vi "Entry.vi"(8 "error in (no error)":errorcluster, 11 "New State":refnum<class "GTH-Assessing.lvclass">) -> (0 "error out":errorcluster, 3 "State out":refnum<class "GTH-Assessing.lvclass">)   [LabVIEW 2014, in "Elevator.lvlib" / "EL-Go To Height.lvlib" / "GTH-Assessing.lvclass"]
doc: "This is an abstract method. Override this method to define the behavior when you enter the state."
uses:
  GTH-Assessing.lvclass
  EL-Go To Height Class/EL-Go To Height.lvclass
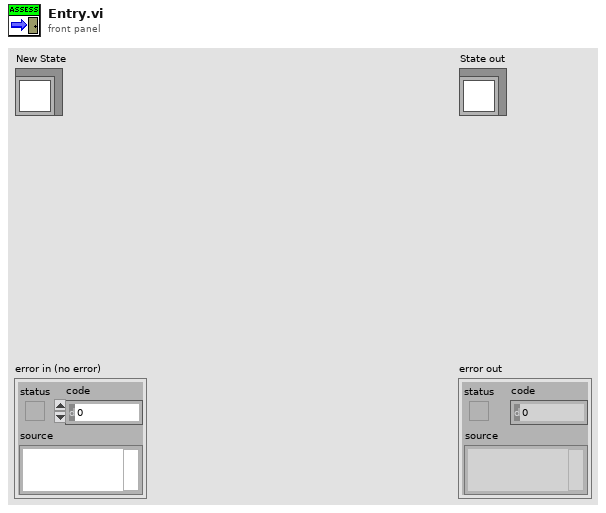
[diagram p1: front panel]
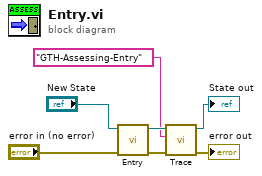
[diagram p0: block diagram]
diagram:
  n1 = call-parent "Entry.vi"("error in (no error)"="error in (no error)", "New State"="New State") -> ("error out"=w5:errorcluster, "State out"=w4:refnum<class "GTH-Assessing.lvclass">)  [unwired: 8 in]
  n2 = call-dynamic "Trace.vi"("error in (no error)"=w5, "Command Action"="GTH-Assessing-Entry", "Command Actor in"=w4) -> ("error out"=→"error out":errorcluster, "Command Actor out"=→"State out":refnum<class "GTH-Assessing.lvclass">)  [unwired: 7 in]
